vi "AT Get Enum Index A.vi"(8 "error in (no error)":errorcluster, 10 "Feature":string, 11 "Handle":i32) -> (0 "error out":errorcluster, 2 "Value":i32, 3 "Status":i32)   [LabVIEW 2019]
doc: "Get Enum Index\n\nOutput:\n I32 Status\n I32 Value\n\nInput:\n I32 Handle\n String Feature\n\nThis function retrieves the currently selected index of the specified enumerated feature. The function will return an error if the feature is currently not readable or if the specified feature is either not an enumerated type feature or is not implemented by the camera."
uses:
  atcoreA.dll
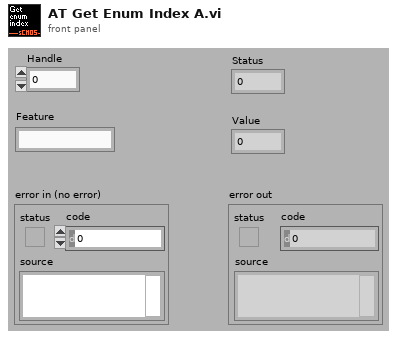
[diagram p1: front panel]
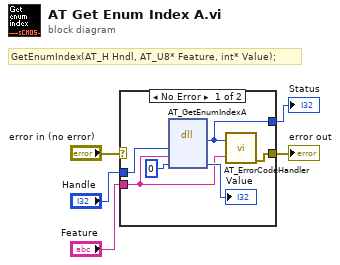
[diagram p0: block diagram]
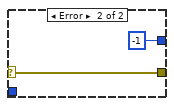
[diagram p2: hidden frame]
diagram:
  # "GetEnumIndex(AT_H Hndl, AT_U8* Feature, int* Value);"
  n1 = case shown="No Error" "error in (no error)" {
    selector: "error in (no error)" -> [_ w13]
    tunnel: [w6 -1] -> w5
    tunnel: "Handle" -> [w11 _]
    tunnel: "Feature" -> [w7 _]
    tunnel: [w8 w13] -> w1
    frame No Error {
      n2 = dll-call lib="atcoreA.dll" fn="AT_GetEnumIndexA"("Handle"=w11, "Feature"=w7, "Value"=0) -> ("Status"=w6:i32, "Value"=→"Value":i32)  [unwired: 5 in, 2 out]
      n3 = call <userlib>:"AT_ErrorCodeHandler.vi"("Error"=w6, "Feature Name"=w7) -> ("error out"=w8:errorcluster)  [unwired: 5 in]
    }
    frame Error {
    }
  }
  "Status" <- w5
  "error out" <- w1
